vi "checkCmd.vi"(8 "error in (no error)":errorcluster, 10 "tcp packet in":string, 11 "tcpServer in":refnum<class "TcpServer.lvclass">) -> (0 "error out":errorcluster, 1 "isCmdRegistered?":bool, 2 "tcp packet out":string, 3 "tcpServer out":refnum<class "TcpServer.lvclass">)   [LabVIEW 2018, in "TcpServer.lvclass"]
doc: "Check if incomming command is in the list of registered commands by the LabVIEW component."
uses:
  TcpServer.lvclass
  TcpServer.lvclass/TcpServer.ctl
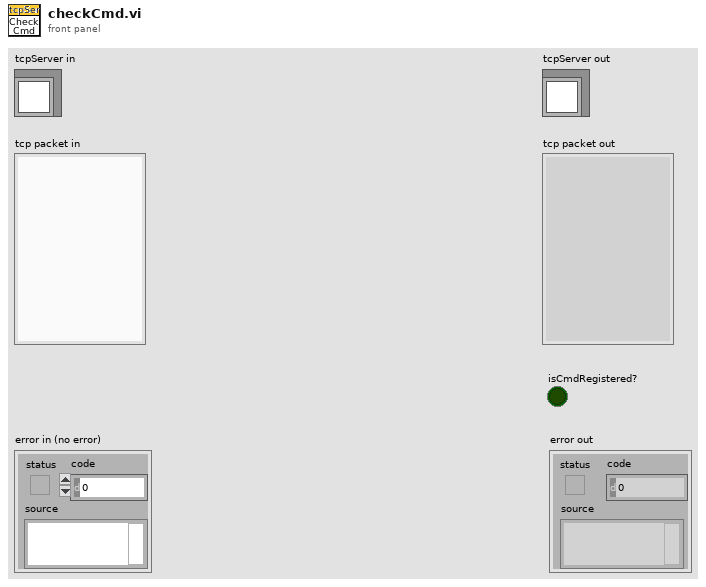
[diagram p1: front panel]
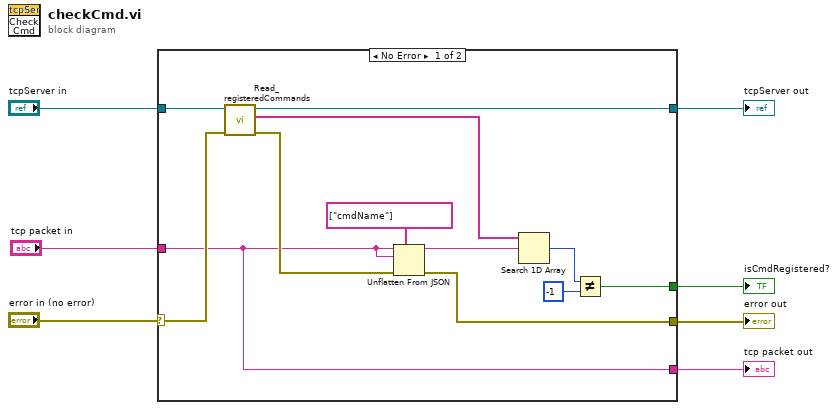
[diagram p0: block diagram]
diagram:
  n1 = case shown="No Error" "error in (no error)" {
    selector: "error in (no error)" -> [w10 w22]
    tunnel: [w14 w22] -> w6
    tunnel: [w11 w21] -> w4
    tunnel: "tcpServer in" -> [w13 w21]
    tunnel: "tcp packet in" -> [w8 w20]
    tunnel: [w17 _] -> w3
    tunnel: [w8 w20] -> w1
    frame No Error {
      n2 = call "Read_registeredCommands.vi"("error in (no error)"=w10, "TcpServer in"=w13) -> ("error out"=w9:errorcluster, "registeredCommands"=w12:string[], "TcpServer out"=w11:refnum<class "TcpServer.lvclass">)  [unwired: 7 in]
      n3 = Unflatten From JSON(path=string[] ["cmdName"] ("tcp packet"), JSON string=w8, type and defaults=w8, error in (no error)=w9) -> (value=w15:string, error out=w14:errorcluster)  [unwired: 3 in]
      n4 = Search 1D Array(1D array=w12, element=w15) -> (index of element=w19:i32)  [unwired: 1 in]
      n5 = Not Equal?(x=w19, y=-1) -> (x != y?=w17:bool)
    }
    frame Error {
    }
  }
  "error out" <- w6
  "tcpServer out" <- w4
  "isCmdRegistered?" <- w3
  "tcp packet out" <- w1
